vi "Process Image.vi"(8 "error in (no error)":errorcluster, 11 "EmbedImage in":refnum<class "EmbedImage.lvclass">) -> (0 "error out":errorcluster, 3 "EmbedImage out":refnum<class "EmbedImage.lvclass">)   [LabVIEW 2023, in "EmbedImage.lvlib" / "EmbedImage.lvclass"]
uses:
  Library/EmbedImage.lvclass
  Custom Controls/Image Types.ctl
  Library/EmbedImage.lvclass/EmbedImage.ctl
panel:
  in  "Image Types":T1
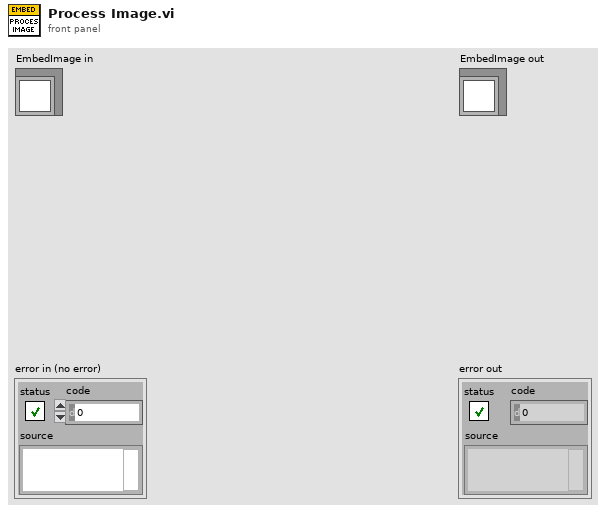
[diagram p1: front panel]
types:
  T1 = typedef "EmbedImage.lvlib/EmbedImage.lvclass/Image Types.ctl" = enum16{"PNG", "JPG", "JPEG", "BMP"}
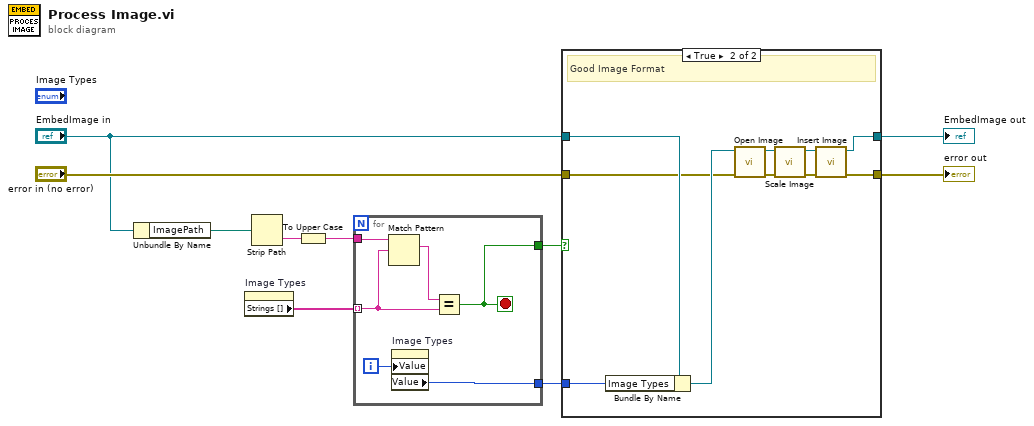
[diagram p0: block diagram]
diagram:
  n1 = Unbundle By Name("EmbedImage in") -> ("ImagePath"=w10:path)
  n2 = property on="Image Types" class="Enum (strict)"() -> ("Strings []"=w7:string[])  [unwired: 2 in, 2 out]
  n3 = Strip Path(path=w10) -> (name=w9:string)  [unwired: 1 out]
  n4 = To Upper Case(1:w9) -> (0:w8:string)
  n5 = for {
    tunnel: w8 -> [w16]
    tunnel: w7 -> [w14] mode=indexing
    tunnel: [w12] -> w4
    tunnel: [w11] -> w2
    i -> [w13]
    stop <- w12 stop-if-true
    n6 = Match Pattern(string=w16, regular expression=w14) -> (match substring=w15:string)  [unwired: 1 in, 3 out]
    n7 = property on="Image Types" class="Enum (strict)"("Value"=w13) -> ("Value"=w11:T1)  [unwired: 2 in, 2 out]
    n8 = Equal?(x=w15, y=w14) -> (x = y?=w12:bool)
  }
  n9 = case shown="True" w4 {
    tunnel: "error in (no error)" -> [w17 w25]
    tunnel: "EmbedImage in" -> [w18 w28]
    tunnel: [w17 w23] -> w3
    tunnel: w2 -> [_ w27]
    tunnel: [w18 w22] -> w1
    frame False {
      # "Unrecognized Image"
    }
    frame True {
      # "Good Image Format"
      n10 = Bundle By Name(cluster=w28, "Image Types"=w27) -> (w26:refnum<class "EmbedImage.lvclass">)
      n11 = call "Open Image.vi"("error in (no error)"=w25, "EmbedImage in"=w26) -> ("error out"=w24:errorcluster, "EmbedImage out"=w20:refnum<class "EmbedImage.lvclass">)  [unwired: 8 in]
      n12 = call "Scale Image.vi"("error in (no error)"=w24, "EmbedImage in"=w20) -> ("error out"=w21:errorcluster, "EmbedImage out"=w19:refnum<class "EmbedImage.lvclass">)  [unwired: 8 in]
      n13 = call "Insert Image.vi"("error in (no error)"=w21, "EmbedImage in"=w19) -> ("error out"=w23:errorcluster, "EmbedImage out"=w22:refnum<class "EmbedImage.lvclass">)  [unwired: 8 in]
    }
  }
  "error out" <- w3
  "EmbedImage out" <- w1
